vi "Condition Tag Names.vi"(11 "tags in":string[](array[string])) -> (3 "tags out":string[](array[string]))   [LabVIEW 2023, in "uLib.lvlib" / "uData.lvclass"]
doc: "Condition the tag name, to make it case insensitive and handle special use cases such as blank strings."
uses:
  uData.lvclass
  Blank Key Reserved String.vi
  uData.lvclass/uData.ctl
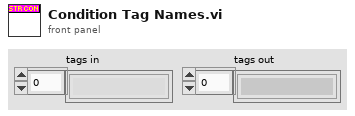
[diagram p1: front panel]
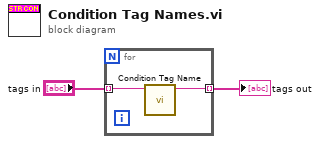
[diagram p0: block diagram]
diagram:
  n1 = for {
    tunnel: "tags in" -> [w4] mode=indexing
    tunnel: [w3] -> w1 mode=indexing
    n2 = call "Condition Tag Name.vi"("tag in"=w4) -> ("tag out"=w3:string)  [unwired: 10 in]
  }
  "tags out" <- w1
